vi "Calibrate P2.vi"(0 "Image In":T1, 2 "Image Type":enum16{"RGB", "Grayscale"}(ring), 11 "Error In":errorcluster, 13 "File Path (Image Calibration P2)":path=path "C:/Users/serce/Desktop/Smart Vision System Testbench/Grid Calibration.png") -> (4 "Corrected Image":T1, 15 "Error Out":errorcluster)   [LabVIEW 2020, in "BilGör.lvlib"]
uses:
  <vilib>/vision/Image Controls.llb/IMAQ Image.ctl
  <vilib>/vision/NI_Vision_Development_Module.lvlib
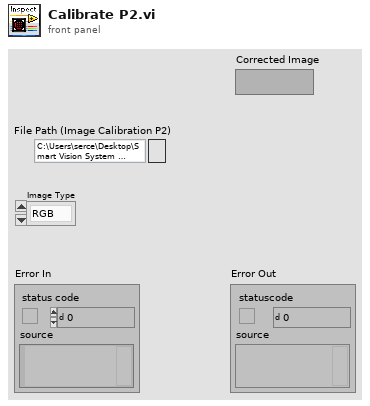
[diagram p1: front panel]
types:
  T1 = typedef "IMAQ Image.ctl" = refnum<image>
  T2 = cluster{"Origin Pixel":cluster{"X":sgl, "Y":sgl}, "X Axis Pixel":cluster{"X":sgl, "Y":sgl}, "Axis Reference":u32}
  T3 = cluster{"Brightness":sgl, "Contrast":sgl, "Gamma":sgl}
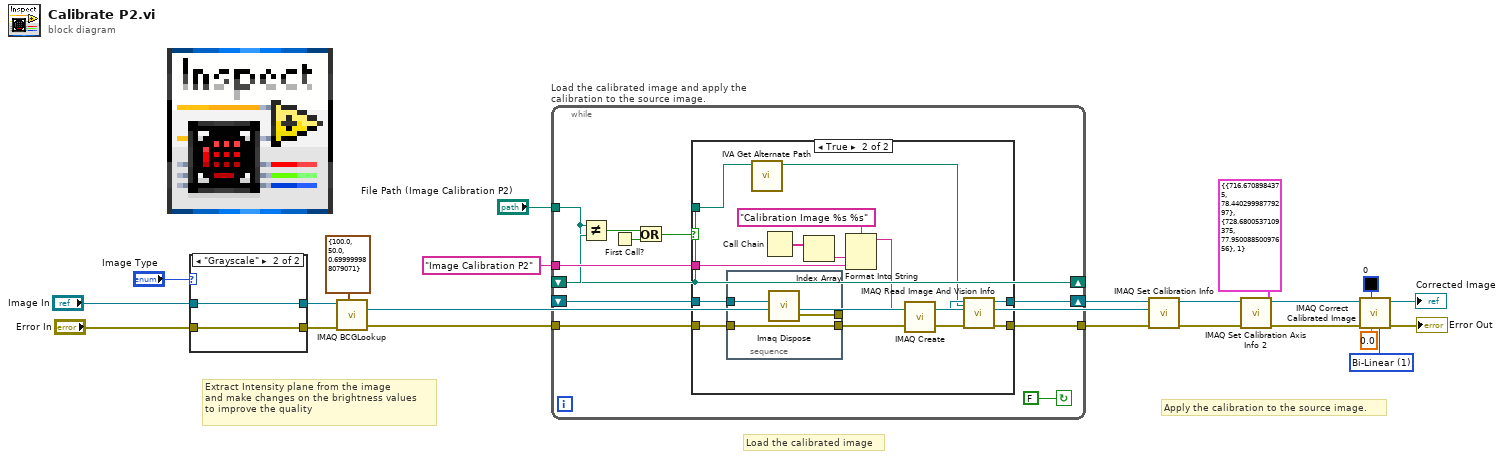
[diagram p0: block diagram]
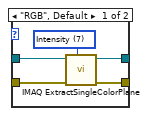
[diagram p2: hidden frame]
diagram:
  w9 = u32 1 items=["Zero Order", "Bi-Linear", "Quadratic", "Cubic Spline"] ("Interpolation Type")
  # "Apply the calibration to the source image."
  # "Load the calibrated image"
  # "Extract Intensity plane from the image\nand make changes on the brightness values\nto improve the quality"
  n1 = case shown="\"Grayscale\"" "Image Type" {
    tunnel: "Image In" -> [w26 w29]
    tunnel: "Error In" -> [w25 w28]
    tunnel: [w24 w29] -> w20
    tunnel: [w23 w28] -> w19
    frame "RGB", Default {
      w27 = 7 items=["Red", "Green", "Blue", "Hue", "Saturation", "Luminance", "Value", "Intensity"] ("Color Plane")
      n2 = call "IMAQ ExtractSingleColorPlane"("Color Plane"=w27, "error in (no error)"=w25, "Image Src"=w26) -> ("error out"=w23:errorcluster, "Image Dst Out"=w24:T1)  [unwired: 1 in, 6 out]
    }
    frame "Grayscale" {
    }
  }
  n3 = call "IMAQ BCGLookup"("Image Src"=w20, "BCG Values"=T3 {"Brightness"=100.0, "Contrast"=50.0, "Gamma"=0.7}, "error in (no error)"=w19) -> ("Image Dst Out"=w13:T1, "error out"=w17:errorcluster)  [unwired: 2 in, 2 out]
  n4 = while "Load the calibrated image and apply the calibration to the source image." {
    shift-right: [w40] -> w15
    shift-left: _ -> [w39]
    tunnel: [w37] -> w14
    tunnel: w17 -> [w36]
    tunnel: "File Path (Image Calibration P2)" -> [w30]
    tunnel: "Image Calibration P2" ("Step Name") -> [w35]
    shift-right: [w30] -> _
    shift-left: _ -> [w31]
    stop <- FALSE continue-if-true
    n5 = Not Equal?(x=w30, y=w31) -> (x != y?=w33:bool)
    n6 = First Call?() -> (First Call?: T/F=w34:bool)
    n7 = Or(x=w33, y=w34) -> (x .or. y?=w32:bool)
    n8 = case shown="True" w32 {
      tunnel: [w42 w54] -> w40
      tunnel: w39 -> [w42 w46]
      tunnel: [w41 w51] -> w37
      tunnel: w36 -> [w41 w47]
      tunnel: w30 -> [_ w44]
      tunnel: w35 -> [_ w48]
      frame False {
      }
      frame True {
        n9 = stacked-sequence {
          tunnel: w47 -> [w58]
          tunnel: w46 -> [w59]
          tunnel: [w58] -> w45
          tunnel: [w57] -> _
          frame #0 {
            n10 = call "Imaq Dispose"("Image"=w59) -> ("error out"=w57:errorcluster)  [unwired: 2 in, 3 out]
          }
        }
        n11 = call <vilib>:"IVA Get Alternate Path.vi"("Path In"=w44) -> ("Path Out"=w43:path)  [unwired: 10 out]
        n12 = Call Chain() -> (call chain=w50:string[])
        n13 = Index Array(array=w50) -> (element=w49:string)  [unwired: 1 in]
        n14 = Format Into String(format string="Calibration Image %s %s" ("Image Name"), w49, w48) -> (resulting string=w56:string)  [unwired: 2 in, 1 out]
        n15 = call "IMAQ Create"("Image Name"=w56, "error in (no error)"=w45) -> ("New Image"=w53:T1, "error out"=w52:errorcluster)  [unwired: 2 in, 1 out]
        n16 = call "IMAQ Read Image And Vision Info"("File Path"=w43, "error in (no error)"=w52, "Image"=w53) -> ("error out"=w51:errorcluster, "Image Out"=w54:T1)  [unwired: 1 in, 6 out]
      }
    }
  }
  n17 = call "IMAQ Set Calibration Info"("error in (no error)"=w14, "Image Dst"=w13, "Image Src"=w15) -> ("error out"=w11:errorcluster, "Calibrated Image"=w4:T1)  [unwired: 1 in, 6 out]
  n18 = call-poly "IMAQ Set Calibration Axis Info 2"("error in (no error)"=w11, "Calibration Axis Info"=T2 {"Origin Pixel"={"X"=716.6709, "Y"=78.4403}, "X Axis Pixel"={"X"=728.68005, "Y"=77.95009}, "Axis Reference"=1}, "Calibration Template Image In"=w4) -> ("error out"=w7:errorcluster, "Calibration Template Image Out"=w8:T1)  [unwired: 7 out]
  n19 = call "IMAQ Correct Calibrated Image"("Interpolation Type"=w9, "Replace Value"=sgl 0.0, "Color Replace Value"=u32 0, "error in (no error)"=w7, "Image Src"=w8) -> ("error out"=→"Error Out":errorcluster, "Corrected Image"=→"Corrected Image":T1)  [unwired: 2 in, 3 out]
